vi "GetProbePlanCoordinates.vi"(8 "Use index as X coord":bool=TRUE, 9 "Probe Card Channels":i32=1) -> (0 "file path":string, 2 "OK?":bool, 3 "Array":T1(array[cluster]))   [LabVIEW 2018] (continued)
\nLabel=Strip\t101\tX=71108.80\ty=-38543.20 \nLabel=Strip\t102\tX=71464.66\ty=-38487.93 \nLabel=Strip\t103\tX=71121.99\ty=-38387.09 \nLabel=Strip\t104\tX=71477.83\ty=-38331.70 \nLabel=Strip\t105\tX=71135.13\ty=-38230.97 \nLabel=Strip\t106\tX=71490.95\ty=-38175.46 \nLabel=Strip\t107\tX=71148.21\ty=-38074.85 \nLabel=Strip\t108\tX=71504.01\ty=-38019.21 \nLabel=Strip\t109\tX=71161.24\ty=-37918.72 \nLabel=Strip\t110\tX=71517.02\ty=-37862.96 \nLabel=Strip\t111\tX=71174.22\ty=-37762.59 \nLabel=Strip\t112\tX=71529.98\ty=-37706.70 \nLabel=Strip\t113\tX=71187.14\ty=-37606.45 \nLabel=Strip\t114\tX=71542.88\ty=-37550.44 \nLabel=Strip\t115\tX=71200.01\ty=-37450.30 \nLabel=Strip\t116\tX=71555.73\ty=-37394.17 \nLabel=Strip\t117\tX=71212.82\ty=-37294.15 \nLabel=Strip\t118\tX=71568.53\ty=-37237.90 \nLabel=Strip\t119\tX=71225.59\ty=-37138.00 \nLabel=Strip\t120\tX=71581.27\ty=-37081.62 \nLabel=Strip\t121\tX=71238.29\ty=-36981.83 \nLabel=Strip\t122\tX=71593.96\ty=-36925.33 \nLabel=Strip\t123\tX=71250.95\ty=-36825.67 \nLabel=Strip\t124\tX=71606.60\ty=-36769.04 \nLabel=Strip\t125\tX=71263.55\ty=-36669.50 \nLabel=Strip\t126\tX=71619.18\ty=-36612.75 \nLabel=Strip\t127\tX=71276.10\ty=-36513.32 \nLabel=Strip\t128\tX=71631.71\ty=-36456.45 \nLabel=Strip\t129\tX=71288.59\ty=-36357.13 \nLabel=Strip\t130\tX=71644.18\ty=-36300.14 \nLabel=Strip\t131\tX=71301.04\ty=-36200.95 \nLabel=Strip\t132\tX=71656.61\ty=-36143.83 \nLabel=Strip\t133\tX=71313.42\ty=-36044.75 \nLabel=Strip\t134\tX=71668.98\ty=-35987.52 \nLabel=Strip\t135\tX=71325.76\ty=-35888.55 \nLabel=Strip\t136\tX=71681.29\ty=-35831.20 \nLabel=Strip\t137\tX=71338.04\ty=-35732.35 \nLabel=Strip\t138\tX=71693.55\ty=-35674.87 \nLabel=Strip\t139\tX=71350.27\ty=-35576.14 \nLabel=Strip\t140\tX=71705.76\ty=-35518.54 \nLabel=Strip\t141\tX=71362.44\ty=-35419.93 \nLabel=Strip\t142\tX=71717.91\ty=-35362.20 \nLabel=Strip\t143\tX=71374.56\ty=-35263.71 \nLabel=Strip\t144\tX=71730.01\ty=-35205.86 \nLabel=Strip\t145\tX=71386.63\ty=-35107.48 \nLabel=Strip\t146\tX=71742.06\ty=-35049.51 \nLabel=Strip\t147\tX=71398.64\ty=-34951.25 \nLabel=Strip\t148\tX=71754.06\ty=-34893.16 \nLabel=Strip\t149\tX=71410.60\ty=-34795.02 \nLabel=Strip\t150\tX=71766.00\ty=-34736.80 \nLabel=Strip\t151\tX=71422.51\ty=-34638.78 \nLabel=Strip\t152\tX=71777.88\ty=-34580.44 \nLabel=Strip\t153\tX=71434.36\ty=-34482.53 \nLabel=Strip\t154\tX=71789.71\ty=-34424.07 \nLabel=Strip\t155\tX=71446.16\ty=-34326.28 \nLabel=Strip\t156\tX=71801.49\ty=-34267.70 \nLabel=Strip\t157\tX=71457.91\ty=-34170.02 \nLabel=Strip\t158\tX=71813.22\ty=-34111.32 \nLabel=Strip\t159\tX=71469.60\ty=-34013.76 \nLabel=Strip\t160\tX=71824.89\ty=-33954.93 \nLabel=Strip\t161\tX=71481.24\ty=-33857.50 \nLabel=Strip\t162\tX=71836.51\ty=-33798.55 \nLabel=Strip\t163\tX=71492.82\ty=-33701.23 \nLabel=Strip\t164\tX=71848.08\ty=-33642.15 \nLabel=Strip\t165\tX=71504.36\ty=-33544.95 \nLabel=Strip\t166\tX=71859.59\ty=-33485.76 \nLabel=Strip\t167\tX=71515.83\ty=-33388.67 \nLabel=Strip\t168\tX=71871.05\ty=-33329.35 \nLabel=Strip\t169\tX=71527.26\ty=-33232.39 \nLabel=Strip\t170\tX=71882.45\ty=-33172.94 \nLabel=Strip\t171\tX=71538.63\ty=-33076.09 \nLabel=Strip\t172\tX=71893.80\ty=-33016.53 \nLabel=Strip\t173\tX=71549.95\ty=-32919.80 \nLabel=Strip\t174\tX=71905.10\ty=-32860.11 \nLabel=Strip\t175\tX=71561.21\ty=-32763.50 \nLabel=Strip\t176\tX=71916.34\ty=-32703.69 \nLabel=Strip\t177\tX=71572.42\ty=-32607.19 \nLabel=Strip\t178\tX=71927.53\ty=-32547.26 \nLabel=Strip\t179\tX=71583.58\ty=-32450.88 \nLabel=Strip\t180\tX=71938.67\ty=-32390.83 \nLabel=Strip\t181\tX=71594.68\ty=-32294.57 \nLabel=Strip\t182\tX=71949.75\ty=-32234.39 \nLabel=Strip\t183\tX=71605.73\ty=-32138.25 \nLabel=Strip\t184\tX=71960.78\ty=-32077.95 \nLabel=Strip\t185\tX=71616.73\ty=-31981.93 \nLabel=Strip\t186\tX=71971.76\ty=-31921.50 \nLabel=Strip\t187\tX=71627.67\ty=-31825.60 \nLabel=Strip\t188\tX=71982.68\ty=-31765.05 \nLabel=Strip\t189\tX=71638.56\ty=-31669.26 \nLabel=Strip\t190\tX=71993.55\ty=-31608.59 \nLabel=Strip\t191\tX=71649.40\ty=-31512.92 \nLabel=Strip\t192\tX=72004.36\ty=-31452.13 \nLabel=Strip\t193\tX=71660.18\ty=-31356.58 \nLabel=Strip\t194\tX=72015.13\ty=-31295.67 \nLabel=Strip\t195\tX=71670.91\ty=-31200.23 \nLabel=Strip\t196\tX=72025.83\ty=-31139.20 \nLabel=Strip\t197\tX=71681.58\ty=-31043.88 \nLabel=Strip\t198\tX=72036.49\ty=-30982.72 \nLabel=Strip\t199\tX=71692.21\ty=-30887.52 \nLabel=Strip\t200\tX=72047.09\ty=-30826.24 \nLabel=Strip\t201\tX=71702.77\ty=-30731.16 \nLabel=Strip\t202\tX=72057.64\ty=-30669.76 \nLabel=Strip\t203\tX=71713.29\ty=-30574.79 \nLabel=Strip\t204\tX=72068.13\ty=-30513.27 \nLabel=Strip\t205\tX=71723.75\ty=-30418.42 \nLabel=Strip\t206\tX=72078.57\ty=-30356.77 \nLabel=Strip\t207\tX=71734.16\ty=-30262.04 \nLabel=Strip\t208\tX=72088.96\ty=-30200.27 \nLabel=Strip\t209\tX=71744.51\ty=-30105.66 \nLabel=Strip\t210\tX=72099.29\ty=-30043.77 \nLabel=Strip\t211\tX=71754.81\ty=-29949.28 \nLabel=Strip\t212\tX=72109.57\ty=-29887.26 \nLabel=Strip\t213\tX=71765.06\ty=-29792.89 \nLabel=Strip\t214\tX=72119.79\ty=-29730.75 \nLabel=Strip\t215\tX=71775.25\ty=-29636.49 \nLabel=Strip\t216\tX=72129.96\ty=-29574.23 \nLabel=Strip\t217\tX=71785.39\ty=-29480.09 \nLabel=Strip\t218\tX=72140.08\ty=-29417.71 \nLabel=Strip\t219\tX=71795.48\ty=-29323.69 \nLabel=Strip\t220\tX=72150.15\ty=-29261.19 \nLabel=Strip\t221\tX=71805.51\ty=-29167.28 \nLabel=Strip\t222\tX=72160.16\ty=-29104.66 \nLabel=Strip\t223\tX=71815.49\ty=-29010.87 \nLabel=Strip\t224\tX=72170.11\ty=-28948.12 \nLabel=Strip\t225\tX=71825.41\ty=-28854.45 \nLabel=Strip\t226\tX=72180.02\ty=-28791.58 \nLabel=Strip\t227\tX=71835.28\ty=-28698.03 \nLabel=Strip\t228\tX=72189.87\ty=-28635.04 \nLabel=Strip\t229\tX=71845.10\ty=-28541.60 \nLabel=Strip\t230\tX=72199.67\ty=-28478.49 \nLabel=Strip\t231\tX=71854.87\ty=-28385.17 \nLabel=Strip\t232\tX=72209.41\ty=-28321.94 \nLabel=Strip\t233\tX=71864.58\ty=-28228.74 \nLabel=Strip\t234\tX=72219.10\ty=-28165.38 \nLabel=Strip\t235\tX=71874.23\ty=-28072.30 \nLabel=Strip\t236\tX=72228.73\ty=-28008.82 \nLabel=Strip\t237\tX=71883.84\ty=-27915.86 \nLabel=Strip\t238\tX=72238.31\ty=-27852.26 \nLabel=Strip\t239\tX=71893.39\ty=-27759.41 \nLabel=Strip\t240\tX=72247.84\ty=-27695.69 \nLabel=Strip\t241\tX=71902.88\ty=-27602.96 \nLabel=Strip\t242\tX=72257.32\ty=-27539.11 \nLabel=Strip\t243\tX=71912.33\ty=-27446.50 \nLabel=Strip\t244\tX=72266.74\ty=-27382.53 \nLabel=Strip\t245\tX=71921.72\ty=-27290.04 \nLabel=Strip\t246\tX=72276.10\ty=-27225.95 \nLabel=Strip\t247\tX=71931.05\ty=-27133.58 \nLabel=Strip\t248\tX=72285.42\ty=-27069.36 \nLabel=Strip\t249\tX=71940.33\ty=-26977.11 \nLabel=Strip\t250\tX=72294.68\ty=-26912.77 \nLabel=Strip\t251\tX=71949.56\ty=-26820.63 \nLabel=Strip\t252\tX=72303.88\ty=-26756.18 \nLabel=Strip\t253\tX=71958.74\ty=-26664.16 \nLabel=Strip\t254\tX=72313.04\ty=-26599.58 \nLabel=Strip\t255\tX=71967.86\ty=-26507.68 \nLabel=Strip\t256\tX=72322.14\ty=-26442.97 \nLabel=Strip\t257\tX=71976.93\ty=-26351.19 \nLabel=Strip\t258\tX=72331.18\ty=-26286.37 \nLabel=Strip\t259\tX=71985.94\ty=-26194.70 \nLabel=Strip\t260\tX=72340.17\ty=-26129.75 \nLabel=Strip\t261\tX=71994.90\ty=-26038.21 \nLabel=Strip\t262\tX=72349.11\ty=-25973.14 \nLabel=Strip\t263\tX=72003.81\ty=-25881.71 \nLabel=Strip\t264\tX=72357.99\ty=-25816.52 \nLabel=Strip\t265\tX=72012.66\ty=-25725.21 \nLabel=Strip\t266\tX=72366.82\ty=-25659.89 \nLabel=Strip\t267\tX=72021.46\ty=-25568.70 \nLabel=Strip\t268\tX=72375.60\ty=-25503.27 \nLabel=Strip\t269\tX=72030.20\ty=-25412.19 \nLabel=Strip\t270\tX=72384.32\ty=-25346.63 \nLabel=Strip\t271\tX=72038.89\ty=-25255.68 \nLabel=Strip\t272\tX=72392.99\ty=-25190.00 \nLabel=Strip\t273\tX=72047.53\ty=-25099.16 \nLabel=Strip\t274\tX=72401.61\ty=-25033.36 \nLabel=Strip\t275\tX=72056.12\ty=-24942.64 \nLabel=Strip\t276\tX=72410.17\ty=-24876.71 \nLabel=Strip\t277\tX=72064.65\ty=-24786.11 \nLabel=Strip\t278\tX=72418.68\ty=-24720.06 \nLabel=Strip\t279\tX=72073.13\ty=-24629.58 \nLabel=Strip\t280\tX=72427.13\ty=-24563.41 \nLabel=Strip\t281\tX=72081.55\ty=-24473.05 \nLabel=Strip\t282\tX=72435.54\ty=-24406.76 \nLabel=Strip\t283\tX=72089.92\ty=-24316.51 \nLabel=Strip\t284\tX=72443.88\ty=-24250.10 \nLabel=Strip\t285\tX=72098.24\ty=-24159.97 \nLabel=Strip\t286\tX=72452.18\ty=-24093.43 \nLabel=Strip\t287\tX=72106.50\ty=-24003.42 \nLabel=Strip\t288\tX=72460.42\ty=-23936.77 \nLabel=Strip\t289\tX=72114.71\ty=-23846.87 \nLabel=Strip\t290\tX=72468.60\ty=-23780.09 \nLabel=Strip\t291\tX=72122.86\ty=-23690.32 \nLabel=Strip\t292\tX=72476.74\ty=-23623.42 \nLabel=Strip\t293\tX=72130.97\ty=-23533.76 \nLabel=Strip\t294\tX=72484.81\ty=-23466.74 \nLabel=Strip\t295\tX=72139.01\ty=-23377.20 \nLabel=Strip\t296\tX=72492.84\ty=-23310.06 \nLabel=Strip\t297\tX=72147.01\ty=-23220.63 \nLabel=Strip\t298\tX=72500.81\ty=-23153.37 \nLabel=Strip\t299\tX=72154.95\ty=-23064.07 \nLabel=Strip\t300\tX=72508.73\ty=-22996.68 \nLabel=Strip\t301\tX=72162.84\ty=-22907.49 \nLabel=Strip\t302\tX=72516.59\ty=-22839.98 \nLabel=Strip\t303\tX=72170.67\ty=-22750.92 \nLabel=Strip\t304\tX=72524.40\ty=-22683.29 \nLabel=Strip\t305\tX=72178.45\ty=-22594.34 \nLabel=Strip\t306\tX=72532.16\ty=-22526.58 \nLabel=Strip\t307\tX=72186.17\ty=-22437.75 \nLabel=Strip\t308\tX=72539.86\ty=-22369.88 \nLabel=Strip\t309\tX=72193.85\ty=-22281.17 \nLabel=Strip\t310\tX=72547.51\ty=-22213.17 \nLabel=Strip\t311\tX=72201.47\ty=-22124.58 \nLabel=Strip\t312\tX=72555.11\ty=-22056.46 \nLabel=Strip\t313\tX=72209.03\ty=-21967.98 \nLabel=Strip\t314\tX=72562.65\ty=-21899.74 \nLabel=Strip\t315\tX=72216.54\ty=-21811.38 \nLabel=Strip\t316\tX=72570.14\ty=-21743.02 \nLabel=Strip\t317\tX=72224.00\ty=-21654.78 \nLabel=Strip\t318\tX=72577.57\ty=-21586.30 \nLabel=Strip\t319\tX=72231.40\ty=-21498.18 \nLabel=Strip\t320\tX=72584.95\ty=-21429.57 \nLabel=Strip\t321\tX=72238.75\ty=-21341.57 \nLabel=Strip\t322\tX=72592.28\ty=-21272.84 \nLabel=Strip\t323\tX=72246.05\ty=-21184.96 \nLabel=Strip\t324\tX=72599.55\ty=-21116.11 \nLabel=Strip\t325\tX=72253.29\ty=-21028.34 \nLabel=Strip\t326\tX=72606.77\ty=-20959.37 \nLabel=Strip\t327\tX=72260.48\ty=-20871.72 \nLabel=Strip\t328\tX=72613.94\ty=-20802.63 \nLabel=Strip\t329\tX=72267.62\ty=-20715.10 \nLabel=Strip\t330\tX=72621.05\ty=-20645.88 \nLabel=Strip\t331\tX=72274.70\ty=-20558.47 \nLabel=Strip\t332\tX=72628.11\ty=-20489.13 \nLabel=Strip\t333\tX=72281.73\ty=-20401.84 \nLabel=Strip\t334\tX=72635.11\ty=-20332.38 \nLabel=Strip\t335\tX=72288.70\ty=-20245.21 \nLabel=Strip\t336\tX=72642.06\ty=-20175.63 \nLabel=Strip\t337\tX=72295.62\ty=-20088.57 \nLabel=Strip\t338\tX=72648.96\ty=-20018.87 \nLabel=Strip\t339\tX=72302.49\ty=-19931.93 \nLabel=Strip\t340\tX=72655.80\ty=-19862.11 \nLabel=Strip\t341\tX=72309.30\ty=-19775.29 \nLabel=Strip\t342\tX=72662.59\ty=-19705.34 \nLabel=Strip\t343\tX=72316.06\ty=-19618.64 \nLabel=Strip\t344\tX=72669.33\ty=-19548.57 \nLabel=Strip\t345\tX=72322.77\ty=-19461.99 \nLabel=Strip\t346\tX=72676.01\ty=-19391.80 \nLabel=Strip\t347\tX=72329.42\ty=-19305.34 \nLabel=Strip\t348\tX=72682.63\ty=-19235.03 \nLabel=Strip\t349\tX=72336.02\ty=-19148.68 \nLabel=Strip\t350\tX=72689.21\ty=-19078.25 \nLabel=Strip\t351\tX=72342.56\ty=-18992.02 \nLabel=Strip\t352\tX=72695.73\ty=-18921.47 \nLabel=Strip\t353\tX=72349.06\ty=-18835.36 \nLabel=Strip\t354\tX=72702.20\ty=-18764.68 \nLabel=Strip\t355\tX=72355.49\ty=-18678.69 \nLabel=Strip\t356\tX=72708.61\ty=-18607.89 \nLabel=Strip\t357\tX=72361.88\ty=-18522.02 \nLabel=Strip\t358\tX=72714.97\ty=-18451.10 \nLabel=Strip\t359\tX=72368.21\ty=-18365.35 \nLabel=Strip\t360\tX=72721.27\ty=-18294.31 \nLabel=Strip\t361\tX=72374.48\ty=-18208.67 \nLabel=Strip\t362\tX=72727.53\ty=-18137.51 \nLabel=Strip\t363\tX=72380.70\ty=-18051.99 \nLabel=Strip\t364\tX=72733.72\ty=-17980.71 \nLabel=Strip\t365\tX=72386.87\ty=-17895.31 \nLabel=Strip\t366\tX=72739.87\ty=-17823.90 \nLabel=Strip\t367\tX=72392.99\ty=-17738.63 \nLabel=Strip\t368\tX=72745.96\ty=-17667.10 \nLabel=Strip\t369\tX=72399.05\ty=-17581.94 \nLabel=Strip\t370\tX=72751.99\ty=-17510.28 \nLabel=Strip\t371\tX=72405.06\ty=-17425.25 \nLabel=Strip\t372\tX=72757.98\ty=-17353.47 \nLabel=Strip\t373\tX=72411.01\ty=-17268.55 \nLabel=Strip\t374\tX=72763.91\ty=-17196.65 \nLabel=Strip\t375\tX=72416.91\ty=-17111.85 \nLabel=Strip\t376\tX=72769.78\ty=-17039.84 \nLabel=Strip\t377\tX=72422.76\ty=-16955.15 \nLabel=Strip\t378\tX=72775.60\ty=-16883.01 \nLabel=Strip\t379\tX=72428.55\ty=-16798.45 \nLabel=Strip\t380\tX=72781.37\ty=-16726.19 \nLabel=Strip\t381\tX=72434.29\ty=-16641.74 \nLabel=Strip\t382\tX=72787.09\ty=-16569.36 \nLabel=Strip\t383\tX=72439.97\ty=-16485.03 \nLabel=Strip\t384\tX=72792.74\ty=-16412.53 \nLabel=Strip\t385\tX=72445.60\ty=-16328.32 \nLabel=Strip\t386\tX=72798.35\ty=-16255.69 \nLabel=Strip\t387\tX=72451.18\ty=-16171.60 \nLabel=Strip\t388\tX=72803.90\ty=-16098.85 \nLabel=Strip\t389\tX=72456.70\ty=-16014.88 \nLabel=Strip\t390\tX=72809.40\ty=-15942.01 \nLabel=Strip\t391\tX=72462.17\ty=-15858.16 \nLabel=Strip\t392\tX=72814.85\ty=-15785.17 \nLabel=Strip\t393\tX=72467.59\ty=-15701.44 \nLabel=Strip\t394\tX=72820.24\ty=-15628.32 \nLabel=Strip\t395\tX=72472.95\ty=-15544.71 \nLabel=Strip\t396\tX=72825.58\ty=-15471.47 \nLabel=Strip\t397\tX=72478.26\ty=-15387.98 \nLabel=Strip\t398\tX=72830.86\ty=-15314.62 \nLabel=Strip\t399\tX=72483.52\ty=-15231.24 \nLabel=Strip\t400\tX=72836.09\ty=-15157.77 \nLabel=Strip\t401\tX=72488.72\ty=-15074.51 \nLabel=Strip\t402\tX=72841.27\ty=-15000.91 \nLabel=Strip\t403\tX=72493.86\ty=-14917.77 \nLabel=Strip\t404\tX=72846.39\ty=-14844.05 \nLabel=Strip\t405\tX=72498.96\ty=-14761.03 \nLabel=Strip\t406\tX=72851.46\ty=-14687.18 \nLabel=Strip\t407\tX=72504.00\ty=-14604.28 \nLabel=Strip\t408\tX=72856.47\ty=-14530.32 \nLabel=Strip\t409\tX=72508.98\ty=-14447.53 \nLabel=Strip\t410\tX=72861.43\ty=-14373.45 \nLabel=Strip\t411\tX=72513.92\ty=-14290.78 \nLabel=Strip\t412\tX=72866.34\ty=-14216.58 \nLabel=Strip\t413\tX=72518.79\ty=-14134.03 \nLabel=Strip\t414\tX=72871.19\ty=-14059.70 \nLabel=Strip\t415\tX=72523.62\ty=-13977.28 \nLabel=Strip\t416\tX=72875.99\ty=-13902.83 \nLabel=Strip\t417\tX=72528.39\ty=-13820.52 \nLabel=Strip\t418\tX=72880.74\ty=-13745.95 \nLabel=Strip\t419\tX=72533.11\ty=-13663.76 \nLabel=Strip\t420\tX=72885.43\ty=-13589.07 \nLabel=Strip\t421\tX=72537.77\ty=-13506.99 \nLabel=Strip\t422\tX=72890.06\ty=-13432.18 \nLabel=Strip\t423\tX=72542.38\ty=-13350.23 \nLabel=Strip\t424\tX=72894.65\ty=-13275.29 \nLabel=Strip\t425\tX=72546.94\ty=-13193.46 \nLabel=Strip\t426\tX=72899.18\ty=-13118.40 \nLabel=Strip\t427\tX=72551.44\ty=-13036.69 \nLabel=Strip\t428\tX=72903.65\ty=-12961.51 \nLabel=Strip\t429\tX=72555.89\ty=-12879.91 \nLabel=Strip\t430\tX=72908.08\ty=-12804.61 \nLabel=Strip\t431\tX=72560.28\ty=-12723.14 \nLabel=Strip\t432\tX=72912.45\ty=-12647.72 \nLabel=Strip\t433\tX=72564.62\ty=-12566.36 \nLabel=Strip\t434\tX=72916.76\ty=-12490.82 \nLabel=Strip\t435\tX=72568.91\ty=-12409.58 \nLabel=Strip\t436\tX=72921.02\ty=-12333.91 \nLabel=Strip\t437\tX=72573.14\ty=-12252.79 \nLabel=Strip\t438\tX=72925.23\ty=-12177.01 \nLabel=Strip\t439\tX=72577.32\ty=-12096.01 \nLabel=Strip\t440\tX=72929.38\ty=-12020.10 \nLabel=Strip\t441\tX=72581.45\ty=-11939.22 \nLabel=Strip\t442\tX=72933.48\ty=-11863.19 \nLabel=Strip\t443\tX=72585.52\ty=-11782.43 \nLabel=Strip\t444\tX=72937.53\ty=-11706.28 \nLabel=Strip\t445\tX=72589.54\ty=-11625.63 \nLabel=Strip\t446\tX=72941.52\ty=-11549.36 \nLabel=Strip\t447\tX=72593.50\ty=-11468.84 \nLabel=Strip\t448\tX=72945.46\ty=-11392.44 \nLabel=Strip\t449\tX=72597.41\ty=-11312.04 \nLabel=Strip\t450\tX=72949.34\ty=-11235.52 \nLabel=Strip\t451\tX=72601.27\ty=-11155.24 \nLabel=Strip\t452\tX=72953.17\ty=-11078.60 \nLabel=Strip\t453\tX=72605.07\ty=-10998.43 \nLabel=Strip\t454\tX=72956.95\ty=-10921.68 \nLabel=Strip\t455\tX=72608.82\ty=-10841.63 \nLabel=Strip\t456\tX=72960.67\ty=-10764.10 \nLabel=Strip\t457\tX=72612.51\ty=-10684.54 \nLabel=Strip\t458\tX=72964.34\ty=-10607.43 \nLabel=Strip\t459\tX=72616.16\ty=-10527.87 \nLabel=Strip\t460\tX=72967.95\ty=-10450.76 \nLabel=Strip\t461\tX=72619.74\ty=-10371.20 \nLabel=Strip\t462\tX=72971.51\ty=-10294.08 \nLabel=Strip\t463\tX=72623.28\ty=-10214.52 \nLabel=Strip\t464\tX=72975.02\ty=-10137.41 \nLabel=Strip\t465\tX=72626.76\ty=-10057.85 \nLabel=Strip\t466\tX=72978.47\ty=-9980.73 \nLabel=Strip\t467\tX=72630.18\ty=-9900.75 \nLabel=Strip\t468\tX=72981.87\ty=-9823.14 \nLabel=Strip\t469\tX=72633.55\ty=-9743.92 \nLabel=Strip\t470\tX=72985.22\ty=-9666.20 \nLabel=Strip\t471\tX=72636.87\ty=-9587.10 \nLabel=Strip\t472\tX=72988.51\ty=-9509.25 \nLabel=Strip\t473\tX=72640.14\ty=-9430.27 \nLabel=Strip\t474\tX=72991.75\ty=-9352.31 \nLabel=Strip\t475\tX=72643.35\ty=-9273.45 \nLabel=Strip\t476\tX=72994.93\ty=-9195.36 \nLabel=Strip\t477\tX=72646.51\ty=-9116.62 \nLabel=Strip\t478\tX=72998.06\ty=-9038.40 \nLabel=Strip\t479\tX=72649.61\ty=-8959.79 \nLabel=Strip\t480\tX=73001.14\ty=-8881.45 \nLabel=Strip\t481\tX=72652.66\ty=-8802.95 \nLabel=Strip\t482\tX=73004.16\ty=-8724.50 \nLabel=Strip\t483\tX=72655.65\ty=-8646.11 \nLabel=Strip\t484\tX=73007.13\ty=-8567.54 \nLabel=Strip\t485\tX=72658.59\ty=-8489.28 \nLabel=Strip\t486\tX=73010.04\ty=-8410.58 \nLabel=Strip\t487\tX=72661.48\ty=-8332.43 \nLabel=Strip\t488\tX=73012.91\ty=-8253.62 \nLabel=Strip\t489\tX=72664.32\ty=-8175.59 \nLabel=Strip\t490\tX=73015.71\ty=-8096.65 \nLabel=Strip\t491\tX=72667.10\ty=-8018.75 \nLabel=Strip\t492\tX=73018.47\ty=-7939.69 \nLabel=Strip\t493\tX=72669.82\ty=-7861.90 \nLabel=Strip\t494\tX=73021.17\ty=-7782.72 \nLabel=Strip\t495\tX=72672.50\ty=-7705.05 \nLabel=Strip\t496\tX=73023.81\ty=-7625.75 \nLabel=Strip\t497\tX=72675.11\ty=-7548.20 \nLabel=Strip\t498\tX=73026.40\ty=-7468.78 \nLabel=Strip\t499\tX=72677.68\ty=-7391.35 \nLabel=Strip\t500\tX=73028.94\ty=-7311.81 \nLabel=Strip\t501\tX=72680.19\ty=-7234.50 \nLabel=Strip\t502\tX=73031.42\ty=-7154.83 \nLabel=Strip\t503\tX=72682.65\ty=-7077.64 \nLabel=Strip\t504\tX=73033.85\ty=-6997.85 \nLabel=Strip\t505\tX=72685.05\ty=-6920.78 \nLabel=Strip\t506\tX=73036.23\ty=-6840.87 \nLabel=Strip\t507\tX=72687.40\ty=-6763.92 \nLabel=Strip\t508\tX=73038.55\ty=-6683.89 \nLabel=Strip\t509\tX=72689.70\ty=-6607.06 \nLabel=Strip\t510\tX=73040.82\ty=-6526.91 \nLabel=Strip\t511\tX=72691.94\ty=-6450.20 \nLabel=Strip\t512\tX=73043.03\ty=-6369.93 \nLabel=Strip\t513\tX=72694.13\ty=-6293.33 \nLabel=Strip\t514\tX=73045.19\ty=-6212.94 \nLabel=Strip\t515\tX=72696.26\ty=-6136.47 \nLabel=Strip\t516\tX=73047.30\ty=-6055.95 \nLabel=Strip\t517\tX=72698.34\ty=-5979.60 \nLabel=Strip\t518\tX=73049.35\ty=-5898.96 \nLabel=Strip\t519\tX=72700.37\ty=-5822.73 \nLabel=Strip\t520\tX=73051.35\ty=-5741.97 \nLabel=Strip\t521\tX=72702.34\ty=-5665.86 \nLabel=Strip\t522\tX=73053.30\ty=-5584.98 \nLabel=Strip\t523\tX=72704.26\ty=-5508.98 \nLabel=Strip\t524\tX=73055.19\ty=-5427.98 \nLabel=Strip\t525\tX=72706.12\ty=-5352.11 \nLabel=Strip\t526\tX=73057.02\ty=-5270.99 \nLabel=Strip\t527\tX=72707.93\ty=-5195.23 \nLabel=Strip\t528\tX=73058.81\ty=-5113.99 \nLabel=Strip\t529\tX=72709.69\ty=-5038.35 \nLabel=Strip\t530\tX=73060.54\ty=-4956.99 \nLabel=Strip\t531\tX=72711.39\ty=-4881.47 \nLabel=Strip\t532\tX=73062.21\ty=-4799.99 \nLabel=Strip\t533\tX=72713.04\ty=-4724.59 \nLabel=Strip\t534\tX=73063.83\ty=-4642.98 \nLabel=Strip\t535\tX=72714.64\ty=-4567.70 \nLabel=Strip\t536\tX=73065.40\ty=-4485.98 \nLabel=Strip\t537\tX=72716.18\ty=-4410.82 \nLabel=Strip\t538\tX=73066.91\ty=-4328.97 \nLabel=Strip\t539\tX=72717.67\ty=-4253.93 \nLabel=Strip\t540\tX=73068.37\ty=-4171.97 \nLabel=Strip\t541\tX=72719.10\ty=-4097.04 \nLabel=Strip\t542\tX=73069.78\ty=-4014.96 \nLabel=Strip\t543\tX=72720.48\ty=-3940.15 \nLabel=Strip\t544\tX=73071.13\ty=-3857.95 \nLabel=Strip\t545\tX=72721.81\ty=-3783.26 \nLabel=Strip\t546\tX=73072.43\ty=-3700.93 \nLabel=Strip\t547\tX=72723.08\ty=-3626.37 \nLabel=Strip\t548\tX=73073.67\ty=-3543.92 \nLabel=Strip\t549\tX=72724.30\ty=-3469.47 \nLabel=Strip\t550\tX=73074.86\ty=-3386.90 \nLabel=Strip\t551\tX=72725.46\ty=-3312.58 \nLabel=Strip\t552\tX=73076.00\ty=-3229.89 \nLabel=Strip\t553\tX=72726.57\ty=-3155.68 \nLabel=Strip\t554\tX=73077.08\ty=-3072.87 \nLabel=Strip\t555\tX=72727.63\ty=-2998.78 \nLabel=Strip\t556\tX=73078.11\ty=-2915.85 \nLabel=Strip\t557\tX=72728.63\ty=-2841.88 \nLabel=Strip\t558\tX=73079.08\ty=-2758.83 \nLabel=Strip\t559\tX=72729.58\ty=-2684.98 \nLabel=Strip\t560\tX=73080.00\ty=-2601.81 \nLabel=Strip\t561\tX=72730.48\ty=-2528.08 \nLabel=Strip\t562\tX=73080.87\ty=-2444.78 \nLabel=Strip\t563\tX=72731.32\ty=-2371.17 \nLabel=Strip\t564\tX=73081.68\ty=-2287.76 \nLabel=Strip\t565\tX=72732.11\ty=-2214.27 \nLabel=Strip\t566\tX=73082.44\ty=-2130.73 \nLabel=Strip\t567\tX=72732.84\ty=-2057.36 \nLabel=Strip\t568\tX=73083.15\ty=-1973.70 \nLabel=Strip\t569\tX=72733.52\ty=-1900.45 \nLabel=Strip\t570\tX=73083.80\ty=-1816.68 \nLabel=Strip\t571\tX=72734.14\ty=-1743.55 \nLabel=Strip\t572\tX=73084.39\ty=-1659.65 \nLabel=Strip\t573\tX=72734.72\ty=-1586.64 \nLabel=Strip\t574\tX=73084.94\ty=-1502.61 \nLabel=Strip\t575\tX=72735.23\ty=-1429.72 \nLabel=Strip\t576\tX=73085.43\ty=-1345.58 \nLabel=Strip\t577\tX=72735.70\ty=-1272.81 \nLabel=Strip\t578\tX=73085.86\ty=-1188.55 \nLabel=Strip\t579\tX=72736.11\ty=-1115.90 \nLabel=Strip\t580\tX=73086.24\ty=-1031.51 \nLabel=Strip\t581\tX=72736.46\ty=-958.98 \nLabel=Strip\t582\tX=73086.57\ty=-874.48 \nLabel=Strip\t583\tX=72736.77\ty=-802.07 \nLabel=Strip\t584\tX=73086.84\ty=-717.44 \nLabel=Strip\t585\tX=72737.02\ty=-645.15 \nLabel=Strip\t586\tX=73087.06\ty=-560.40 \nLabel=Strip\t587\tX=72737.21\ty=-488.23 \nLabel=Strip\t588\tX=73087.23\ty=-403.36 \nLabel=Strip\t589\tX=72737.35\ty=-331.31 \nLabel=Strip\t590\tX=73087.34\ty=-246.32 \nLabel=Strip\t591\tX=72737.44\ty=-174.39 \nLabel=Strip\t592\tX=73087.40\ty=-89.28 \nLabel=Strip\t593\tX=72737.47\ty=-17.47 \nLabel=Strip\t594\tX=73087.40\ty=67.76 \nLabel=Strip\t595\tX=72737.45\ty=139.46 \nLabel=Strip\t596\tX=73087.35\ty=224.80 \nLabel=Strip\t597\tX=72737.38\ty=296.38 \nLabel=Strip\t598\tX=73087.25\ty=381.85 \nLabel=Strip\t599\tX=72737.25\ty=453.31 \nLabel=Strip\t600\tX=73087.09\ty=538.89 \nLabel=Strip\t601\tX=72737.06\ty=610.23 \nLabel=Strip\t602\tX=73086.88\ty=695.94 \nLabel=Strip\t603\tX=72736.83\ty=767.16 \nLabel=Strip\t604\tX=73086.61\ty=852.99 \nLabel=Strip\t605\tX=72736.54\ty=924.09 \nLabel=Strip\t606\tX=73086.29\ty=1010.04 \nLabel=Strip\t607\tX=72736.19\ty=1081.01 \nLabel=Strip\t608\tX=73085.92\ty=1167.09 \nLabel=Strip\t609\tX=72735.79\ty=1237.94 \nLabel=Strip\t610\tX=73085.49\ty=1324.14 \nLabel=Strip\t611\tX=72735.34\ty=1394.87 \nLabel=Strip\t612\tX=73085.01\ty=1481.19 \nLabel=Strip\t613\tX=72734.84\ty=1551.81 \nLabel=Strip\t614\tX=73084.47\ty=1638.24 \nLabel=Strip\t615\tX=72734.28\ty=1708.74 \nLabel=Strip\t616\tX=73083.88\ty=1795.29 \nLabel=Strip\t617\tX=72733.66\ty=1865.67 \nLabel=Strip\t618\tX=73083.24\ty=1952.35 \nLabel=Strip\t619\tX=72733.00\ty=2022.60 \nLabel=Strip\t620\tX=73082.54\ty=2109.40 \nLabel=Strip\t621\tX=72732.27\ty=2179.54 \nLabel=Strip\t622\tX=73081.79\ty=2266.45 \nLabel=Strip\t623\tX=72731.50\ty=2336.47 \nLabel=Strip\t624\tX=73080.98\ty=2423.51 \nLabel=Strip\t625\tX=72730.67\ty=2493.41 \nLabel=Strip\t626\tX=73080.13\ty=2580.57 \nLabel=Strip\t627\tX=72729.78\ty=2650.35 \nLabel=Strip\t628\tX=73079.21\ty=2737.62 \nLabel=Strip\t629\tX=72728.85\ty=2807.29 \nLabel=Strip\t630\tX=73078.24\ty=2894.68 \nLabel=Strip\t631\tX=72727.86\ty=2964.22 \nLabel=Strip\t632\tX=73077.22\ty=3051.74 \nLabel=Strip\t633\tX=72726.81\ty=3121.16 \nLabel=Strip\t634\tX=73076.15\ty=3208.80 \nLabel=Strip\t635\tX=72725.71\ty=3278.10 \nLabel=Strip\t636\tX=73075.02\ty=3365.86 \nLabel=Strip\t637\tX=72724.56\ty=3435.04 \nLabel=Strip\t638\tX=73073.84\ty=3522.92 \nLabel=Strip\t639\tX=72723.35\ty=3591.98 \nLabel=Strip\t640\tX=73072.60\ty=3679.98 \nLabel=Strip\t641\tX=72722.09\ty=3748.93 \nLabel=Strip\t642\tX=73071.31\ty=3837.05 \nLabel=Strip\t643\tX=72720.78\ty=3905.87 \nLabel=Strip\t644\tX=73069.96\ty=3994.11 \nLabel=Strip\t645\tX=72719.41\ty=4062.81 \nLabel=Strip\t646\tX=73068.56\ty=4151.17 \nLabel=Strip\t647\tX=72717.99\ty=4219.75 \nLabel=Strip\t648\tX=73067.11\ty=4308.23 \nLabel=Strip\t649\tX=72716.51\ty=4376.70 \nLabel=Strip\t650\tX=73065.60\ty=4465.30 \nLabel=Strip\t651\tX=72714.98\ty=4533.64 \nLabel=Strip\t652\tX=73064.04\ty=4622.36 \nLabel=Strip\t653\tX=72713.39\ty=4690.59 \nLabel=Strip\t654\tX=73062.43\ty=4779.43 \nLabel=Strip\t655\tX=72711.76\ty=4847.53 \nLabel=Strip\t656\tX=73060.76\ty=4936.49 \nLabel=Strip\t657\tX=72710.06\ty=5004.48 \nLabel=Strip\t658\tX=73059.04\ty=5093.56 \nLabel=Strip\t659\tX=72708.32\ty=5161.42 \nLabel=Strip\t660\tX=73057.26\ty=5250.63 \nLabel=Strip\t661\tX=72706.52\ty=5318.37 \nLabel=Strip\t662\tX=73055.43\ty=5407.69 \nLabel=Strip\t663\tX=72704.66\ty=5475.32 \nLabel=Strip\t664\tX=73053.54\ty=5564.76 \nLabel=Strip\t665\tX=72702.76\ty=5632.27 \nLabel=Strip\t666\tX=73051.61\ty=5721.83 \nLabel=Strip\t667\tX=72700.79\ty=5789.21 \nLabel=Strip\t668\tX=73049.61\ty=5878.90 \nLabel=Strip\t669\tX=72698.78\ty=5946.16 \nLabel=Strip\t670\tX=73047.57\ty=6035.97 \nLabel=Strip\t671\tX=72696.71\ty=6103.11 \nLabel=Strip\t672\tX=73045.47\ty=6193.04 \nLabel=Strip\t673\tX=72694.58\ty=6260.06 \nLabel=Strip\t674\tX=73043.31\ty=6350.10 \nLabel=Strip\t675\tX=72692.41\ty=6417.01 \nLabel=Strip\t676\tX=73041.10\ty=6507.17 \nLabel=Strip\t677\tX=72690.18\ty=6573.96 \nLabel=Strip\t678\tX=73038.84\ty=6664.24 \nLabel=Strip\t679\tX=72687.89\ty=6730.91 \nLabel=Strip\t680\tX=73036.52\ty=6821.31 \nLabel=Strip\t681\tX=72685.55\ty=6887.86 \nLabel=Strip\t682\tX=73034.15\ty=6978.38 \nLabel=Strip\t683\tX=72683.16\ty=7044.81 \nLabel=Strip\t684\tX=73031.73\ty=7135.45 \nLabel=Strip\t685\tX=72680.71\ty=7201.76 \nLabel=Strip\t686\tX=73029.25\ty=7292.52 \nLabel=Strip\t687\tX=72678.21\ty=7358.71 \nLabel=Strip\t688\tX=73026.72\ty=7449.59 \nLabel=Strip\t689\tX=72675.65\ty=7515.66 \nLabel=Strip\t690\tX=73024.13\ty=7606.67 \nLabel=Strip\t691\tX=72673.04\ty=7672.61 \nLabel=Strip\t692\tX=73021.49\ty=7763.74 \nLabel=Strip\t693\tX=72670.38\ty=7829.56 \nLabel=Strip\t694\tX=73018.80\ty=7920.81 \nLabel=Strip\t695\tX=72667.67\ty=7986.51 \nLabel=Strip\t696\tX=73016.05\ty=8077.88 \nLabel=Strip\t697\tX=72664.89\ty=8143.46 \nLabel=Strip\t698\tX=73013.25\ty=8234.95 \nLabel=Strip\t699\tX=72662.07\ty=8300.41 \nLabel=Strip\t700\tX=73010.39\ty=8392.02 \nLabel=Strip\t701\tX=72659.19\ty=8457.36 \nLabel=Strip\t702\tX=73007.48\ty=8549.09 \nLabel=Strip\t703\tX=72656.26\ty=8614.32 \nLabel=Strip\t704\tX=73004.52\ty=8706.16 \nLabel=Strip\t705\tX=72653.27\ty=8771.27 \nLabel=Strip\t706\tX=73001.50\ty=8863.24 \nLabel=Strip\t707\tX=72650.23\ty=8928.22 \nLabel=Strip\t708\tX=72998.42\ty=9020.31 \nLabel=Strip\t709\tX=72647.14\ty=9085.17 \nLabel=Strip\t710\tX=72995.30\ty=9177.38 \nLabel=Strip\t711\tX=72643.99\ty=9242.12 \nLabel=Strip\t712\tX=72992.12\ty=9334.45 \nLabel=Strip\t713\tX=72640.78\ty=9399.07 \nLabel=Strip\t714\tX=72988.88\ty=9491.52 \nLabel=Strip\t715\tX=72637.53\ty=9556.02 \nLabel=Strip\t716\tX=72985.60\ty=9648.59 \nLabel=Strip\t717\tX=72634.22\ty=9712.97 \nLabel=Strip\t718\tX=72982.25\ty=9805.66 \nLabel=Strip\t719\tX=72630.85\ty=9869.92 \nLabel=Strip\t720\tX=72978.86\ty=9962.73 \nLabel=Strip\t721\tX=72627.43\ty=10026.88 \nLabel=Strip\t722\tX=72975.41\ty=10119.81 \nLabel=Strip\t723\tX=72623.96\ty=10183.83 \nLabel=Strip\t724\tX=72971.90\ty=10276.88 \nLabel=Strip\t725\tX=72620.44\ty=10340.78 \nLabel=Strip\t726\tX=72968.34\ty=10433.95 \nLabel=Strip\t727\tX=72616.86\ty=10497.73 \nLabel=Strip\t728\tX=72964.73\ty=10591.02 \nLabel=Strip\t729\tX=72613.22\ty=10654.68 \nLabel=Strip\t730\tX=72961.07\ty=10748.09 \nLabel=Strip\t731\tX=72609.53\ty=10811.63 \nLabel=Strip\t732\tX=72957.35\ty=10905.16 \nLabel=Strip\t733\tX=72605.79\ty=10968.58 \nLabel=Strip\t734\tX=72953.57\ty=11062.23 \nLabel=Strip\t735\tX=72602.00\ty=11125.53 \nLabel=Strip\t736\tX=72949.74\ty=11219.29 \nLabel=Strip\t737\tX=72598.15\ty=11282.48 \nLabel=Strip\t738\tX=72945.86\ty=11376.36 \nLabel=Strip\t739\tX=72594.24\ty=11439.42 \nLabel=Strip\t740\tX=72941.93\ty=11533.43 \nLabel=Strip\t741\tX=72590.28\ty=11596.37 \nLabel=Strip\t742\tX=72937.94\ty=11690.50 \nLabel=Strip\t743\tX=72586.27\ty=11753.32 \nLabel=Strip\t744\tX=72933.89\ty=11847.57 \nLabel=Strip\t745\tX=72582.21\ty=11910.27 \nLabel=Strip\t746\tX=72929.79\ty=12004.64 \nLabel=Strip\t747\tX=72578.09\ty=12067.22 \nLabel=Strip\t748\tX=72925.64\ty=12161.70 \nLabel=Strip\t749\tX=72573.91\ty=12224.16 \nLabel=Strip\t750\tX=72921.43\ty=12318.77 \nLabel=Strip\t751\tX=72569.69\ty=12381.11 \nLabel=Strip\t752\tX=72917.17\ty=12475.84 \nLabel=Strip\t753\tX=72565.41\ty=12538.06 \nLabel=Strip\t754\tX=72912.86\ty=12632.90 \nLabel=Strip\t755\tX=72561.07\ty=12695.00 \nLabel=Strip\t756\tX=72908.49\ty=12789.97 \nLabel=Strip\t757\tX=72556.68\ty=12851.95 \nLabel=Strip\t758\tX=72904.07\ty=12947.03 \nLabel=Strip\t759\tX=72552.24\ty=13008.89 \nLabel=Strip\t760\tX=72899.59\ty=13104.10 \nLabel=Strip\t761\tX=72547.74\ty=13165.84 \nLabel=Strip\t762\tX=72895.06\ty=13261.16 \nLabel=Strip\t763\tX=72543.19\ty=13322.78 \nLabel=Strip\t764\tX=72890.48\ty=13418.23 \nLabel=Strip\t765\tX=72538.58\ty=13479.72 \nLabel=Strip\t766\tX=72885.84\ty=13575.29 \nLabel=Strip\t767\tX=72533.92\ty=13636.67 \nLabel=Strip\t768\tX=72881.15\ty=13732.35 \nLabel=Strip\t769\tX=72529.21\ty=13793.61 \nLabel=Strip\t770\tX=72876.40\ty=13889.41 \nLabel=Strip\t771\tX=72524.44\ty=13950.55 \nLabel=Strip\t772\tX=72871.60\ty=14046.47 \nLabel=Strip\t773\tX=72519.62\ty=14107.49 \nLabel=Strip\t774\tX=72866.75\ty=14203.53 \nLabel=Strip\t775\tX=72514.75\ty=14264.43 \nLabel=Strip\t776\tX=72861.84\ty=14360.59 \nLabel=Strip\t777\tX=72509.82\ty=14421.37 \nLabel=Strip\t778\tX=72856.88\ty=14517.65 \nLabel=Strip\t779\tX=72504.83\ty=14578.31 \nLabel=Strip\t780\tX=72851.86\ty=14674.71 \nLabel=Strip\t781\tX=72499.80\ty=14735.25 \nLabel=Strip\t782\tX=72846.79\ty=14831.77 \nLabel=Strip\t783\tX=72494.71\ty=14892.18 \nLabel=Strip\t784\tX=72841.67\ty=14988.83 \nLabel=Strip\t785\tX=72489.56\ty=15049.12 \nLabel=Strip\t786\tX=72836.49\ty=15145.88 \nLabel=Strip\t787\tX=72484.36\ty=15206.06 \nLabel=Strip\t788\tX=72831.26\ty=15302.94 \nLabel=Strip\t789\tX=72479.11\ty=15362.99 \nLabel=Strip\t790\tX=72825.97\ty=15459.99 \nLabel=Strip\t791\tX=72473.80\ty=15519.93 \nLabel=Strip\t792\tX=72820.63\ty=15617.05 \nLabel=Strip\t793\tX=72468.44\ty=15676.86 \nLabel=Strip\t794\tX=72815.24\ty=15774.10 \nLabel=Strip\t795\tX=72463.03\ty=15833.79 \nLabel=Strip\t796\tX=72809.79\ty=15931.15 \nLabel=Strip\t797\tX=72457.56\ty=15990.72 \nLabel=Strip\t798\tX=72804.29\ty=16088.21 \nLabel=Strip\t799\tX=72452.03\ty=16147.66 \nLabel=Strip\t800\tX=72798.73\ty=16245.26 \nLabel=Strip\t801\tX=72446.46\ty=16304.59 \nLabel=Strip\t802\tX=72793.12\ty=16402.31 \nLabel=Strip\t803\tX=72440.83\ty=16461.52 \nLabel=Strip\t804\tX=72787.45\ty=16559.36 \nLabel=Strip\t805\tX=72435.14\ty=16618.44 \nLabel=Strip\t806\tX=72781.74\ty=16716.40 \nLabel=Strip\t807\tX=72429.40\ty=16775.37 \nLabel=Strip\t808\tX=72775.96\ty=16873.45 \nLabel=Strip\t809\tX=72423.61\ty=16932.30 \nLabel=Strip\t810\tX=72770.14\ty=17030.50 \nLabel=Strip\t811\tX=72417.76\ty=17089.22 \nLabel=Strip\t812\tX=72764.26\ty=17187.54 \nLabel=Strip\t813\tX=72411.86\ty=17246.15 \nLabel=Strip\t814\tX=72758.32\ty=17344.59 \nLabel=Strip\t815\tX=72405.91\ty=17403.07 \nLabel=Strip\t816\tX=72752.33\ty=17501.63 \nLabel=Strip\t817\tX=72399.90\ty=17559.99 \nLabel=Strip\t818\tX=72746.29\ty=17658.67 \nLabel=Strip\t819\tX=72393.84\ty=17716.92 \nLabel=Strip\t820\tX=72740.19\ty=17815.71 \nLabel=Strip\t821\tX=72387.72\ty=17873.84 \nLabel=Strip\t822\tX=72734.04\ty=17972.75 \nLabel=Strip\t823\tX=72381.55\ty=18030.76 \nLabel=Strip\t824\tX=72727.84\ty=18129.79 \nLabel=Strip\t825\tX=72375.33\ty=18187.67 \nLabel=Strip\t826\tX=72721.58\ty=18286.83 \nLabel=Strip\t827\tX=72369.05\ty=18344.59 \nLabel=Strip\t828\tX=72715.27\ty=18443.87 \nLabel=Strip\t829\tX=72362.72\ty=18501.51 \nLabel=Strip\t830\tX=72708.90\ty=18600.90 \nLabel=Strip\t831\tX=72356.33\ty=18658.42 \nLabel=Strip\t832\tX=72702.48\ty=18757.93 \nLabel=Strip\t833\tX=72349.89\ty=18815.34 \nLabel=Strip\t834\tX=72696.01\ty=18914.97 \nLabel=Strip\t835\tX=72343.39\ty=18972.25 \nLabel=Strip\t836\tX=72689.48\ty=19072.00 \nLabel=Strip\t837\tX=72336.85\ty=19129.16 \nLabel=Strip\t838\tX=72682.90\ty=19229.03 \nLabel=Strip\t839\tX=72330.24\ty=19286.07 \nLabel=Strip\t840\tX=72676.26\ty=19386.06 \nLabel=Strip\t841\tX=72323.59\ty=19442.98 \nLabel=Strip\t842\tX=72669.57\ty=19543.09 \nLabel=Strip\t843\tX=72316.88\ty=19599.89 \nLabel=Strip\t844\tX=72662.82\ty=19700.12 \nLabel=Strip\t845\tX=72310.11\ty=19756.79 \nLabel=Strip\t846\tX=72656.03\ty=19857.14 \nLabel=Strip\t847\tX=72303.29\ty=19913.70 \nLabel=Strip\t848\tX=72649.17\ty=20014.17 \nLabel=Strip\t849\tX=72296.42\ty=20070.60 \nLabel=Strip\t850\tX=72642.27\ty=20171.19 \nLabel=Strip\t851\tX=72289.50\ty=20227.50 \nLabel=Strip\t852\tX=72635.30\ty=20328.21 \nLabel=Strip\t853\tX=72282.52\ty=20384.41 \nLabel=Strip\t854\tX=72628.29\ty=20485.23 \nLabel=Strip\t855\tX=72275.48\ty=20541.31 \nLabel=Strip\t856\tX=72621.22\ty=20642.25 \nLabel=Strip\t857\tX=72268.39\ty=20698.20 \nLabel=Strip\t858\tX=72614.10\ty=20799.27 \nLabel=Strip\t859\tX=72261.25\ty=20855.10 \nLabel=Strip\t860\tX=72606.92\ty=20956.28 \nLabel=Strip\t861\tX=72254.06\ty=21012.00 \nLabel=Strip\t862\tX=72599.69\ty=21113.30 \nLabel=Strip\t863\tX=72246.81\ty=21168.89 \nLabel=Strip\t864\tX=72592.41\ty=21270.31 \nLabel=Strip\t865\tX=72239.50\ty=21325.78 \nLabel=Strip\t866\tX=72585.07\ty=21427.32 \nLabel=Strip\t867\tX=72232.14\ty=21482.67 \nLabel=Strip\t868\tX=72577.67\ty=21584.33 \nLabel=Strip\t869\tX=72224.73\ty=21639.56 \nLabel=Strip\t870\tX=72570.23\ty=21741.34 \nLabel=Strip\t871\tX=72217.27\ty=21796.45 \nLabel=Strip\t872\tX=72562.73\ty=21898.35 \nLabel=Strip\t873\tX=72209.75\ty=21953.34 \nLabel=Strip\t874\tX=72555.17\ty=22055.35 \nLabel=Strip\t875\tX=72202.17\ty=22110.22 \nLabel=Strip\t876\tX=72547.56\ty=22212.36 \nLabel=Strip\t877\tX=72194.54\ty=22267.11 \nLabel=Strip\t878\tX=72539.90\ty=22369.36 \nLabel=Strip\t879\tX=72186.86\ty=22423.99 \nLabel=Strip\t880\tX=72532.18\ty=22526.36 \nLabel=Strip\t881\tX=72179.13\ty=22580.87 \nLabel=Strip\t882\tX=72524.41\ty=22683.36 \nLabel=Strip\t883\tX=72171.34\ty=22737.75 \nLabel=Strip\t884\tX=72516.58\ty=22840.36 \nLabel=Strip\t885\tX=72163.49\ty=22894.62 \nLabel=Strip\t886\tX=72508.70\ty=22997.35 \nLabel=Strip\t887\tX=72155.59\ty=23051.50 \nLabel=Strip\t888\tX=72500.77\ty=23154.35 \nLabel=Strip\t889\tX=72147.64\ty=23208.37 \nLabel=Strip\t890\tX=72492.78\ty=23311.34 \nLabel=Strip\t891\tX=72139.64\ty=23365.24 \nLabel=Strip\t892\tX=72484.74\ty=23468.33 \nLabel=Strip\t893\tX=72131.58\ty=23522.11 \nLabel=Strip\t894\tX=72476.65\ty=23625.32 \nLabel=Strip\t895\tX=72123.46\ty=23678.98 \nLabel=Strip\t896\tX=72468.50\ty=23782.31 \nLabel=Strip\t897\tX=72115.29\ty=23835.85 \nLabel=Strip\t898\tX=72460.30\ty=23939.29 \nLabel=Strip\t899\tX=72107.07\ty=23992.71 \nLabel=Strip\t900\tX=72452.04\ty=24096.28 \nLabel=Strip\t901\tX=72098.80\ty=24149.57 \nLabel=Strip\t902\tX=72443.73\ty=24253.26 \nLabel=Strip\t903\tX=72090.47\ty=24306.44 \nLabel=Strip\t904\tX=72435.36\ty=24410.24 \nLabel=Strip\t905\tX=72082.08\ty=24463.29 \nLabel=Strip\t906\tX=72426.94\ty=24567.22 \nLabel=Strip\t907\tX=72073.65\ty=24620.15 \nLabel=Strip\t908\tX=72418.47\ty=24724.19 \nLabel=Strip\t909\tX=72065.15\ty=24777.01 \nLabel=Strip\t910\tX=72409.94\ty=24881.17 \nLabel=Strip\t911\tX=72056.61\ty=24933.86 \nLabel=Strip\t912\tX=72401.36\ty=25038.14 \nLabel=Strip\t913\tX=72048.01\ty=25090.71 \nLabel=Strip\t914\tX=72392.72\ty=25195.11 \nLabel=Strip\t915\tX=72039.36\ty=25247.56 \nLabel=Strip\t916\tX=72384.03\ty=25352.08 \nLabel=Strip\t917\tX=72030.65\ty=25404.41 \nLabel=Strip\t918\tX=72375.29\ty=25509.04 \nLabel=Strip\t919\tX=72021.88\ty=25561.26 \nLabel=Strip\t920\tX=72366.49\ty=25666.01 \nLabel=Strip\t921\tX=72013.07\ty=25718.10 \nLabel=Strip\t922\tX=72357.64\ty=25822.97 \nLabel=Strip\t923\tX=72004.20\ty=25874.94 \nLabel=Strip\t924\tX=72348.74\ty=25979.93 \nLabel=Strip\t925\tX=71995.28\ty=26031.78 \nLabel=Strip\t926\tX=72339.77\ty=26136.89 \nLabel=Strip\t927\tX=71986.30\ty=26188.62 \nLabel=Strip\t928\tX=72330.76\ty=26293.85 \nLabel=Strip\t929\tX=71977.27\ty=26345.45 \nLabel=Strip\t930\tX=72321.69\ty=26450.80 \nLabel=Strip\t931\tX=71968.18\ty=26502.29 \nLabel=Strip\t932\tX=72312.57\ty=26607.75 \nLabel=Strip\t933\tX=71959.04\ty=26659.12 \nLabel=Strip\t934\tX=72303.40\ty=26764.70 \nLabel=Strip\t935\tX=71949.85\ty=26815.95 \nLabel=Strip\t936\tX=72294.17\ty=26921.65 \nLabel=Strip\t937\tX=71940.60\ty=26972.78 \nLabel=Strip\t938\tX=72284.88\ty=27078.60 \nLabel=Strip\t939\tX=71931.30\ty=27129.60 \nLabel=Strip\t940\tX=72275.54\ty=27235.54 \nLabel=Strip\t941\tX=71921.94\ty=27286.42 \nLabel=Strip\t942\tX=72266.15\ty=27392.48 \nLabel=Strip\t943\tX=71912.53\ty=27443.24 \nLabel=Strip\t944\tX=72256.71\ty=27549.42 \nLabel=Strip\t945\tX=71903.07\ty=27600.06 \nLabel=Strip\t946\tX=72247.21\ty=27706.36 \nLabel=Strip\t947\tX=71893.55\ty=27756.88 \nLabel=Strip\t948\tX=72237.65\ty=27863.29 \nLabel=Strip\t949\tX=71883.98\ty=27913.69 \nLabel=Strip\t950\tX=72228.04\ty=28020.23 \nLabel=Strip\t951\tX=71874.36\ty=28070.50 \nLabel=Strip\t952\tX=72218.38\ty=28177.16 \nLabel=Strip\t953\tX=71864.68\ty=28227.31 \nLabel=Strip\t954\tX=72208.67\ty=28334.09 \nLabel=Strip\t955\tX=71854.94\ty=28384.12 \nLabel=Strip\t956\tX=72198.90\ty=28491.01 \nLabel=Strip\t957\tX=71845.16\ty=28540.92 \nLabel=Strip\t958\tX=72189.07\ty=28647.93 \nLabel=Strip\t959\tX=71835.31\ty=28697.73 \nLabel=Strip\t960\tX=72179.19\ty=28804.85 \nLabel=Strip\t961\tX=71825.42\ty=28854.53 \nLabel=Strip\t962\tX=72169.26\ty=28961.77 \nLabel=Strip\t963\tX=71815.47\ty=29011.32 \nLabel=Strip\t964\tX=72159.27\ty=29118.69 \nLabel=Strip\t965\tX=71805.47\ty=29168.12 \nLabel=Strip\t966\tX=72149.23\ty=29275.60 \nLabel=Strip\t967\tX=71795.41\ty=29324.91 \nLabel=Strip\t968\tX=72139.14\ty=29432.51 \nLabel=Strip\t969\tX=71785.30\ty=29481.70 \nLabel=Strip\t970\tX=72128.99\ty=29589.42 \nLabel=Strip\t971\tX=71775.13\ty=29638.49 \nLabel=Strip\t972\tX=72118.79\ty=29746.33 \nLabel=Strip\t973\tX=71764.91\ty=29795.28 \nLabel=Strip\t974\tX=72108.53\ty=29903.23 \nLabel=Strip\t975\tX=71754.64\ty=29952.06 \nLabel=Strip\t976\tX=72098.22\ty=30060.14 \nLabel=Strip\t977\tX=71744.31\ty=30108.84 \nLabel=Strip\t978\tX=72087.86\ty=30217.03 \nLabel=Strip\t979\tX=71733.93\ty=30265.62 \nLabel=Strip\t980\tX=72077.44\ty=30373.93 \nLabel=Strip\t981\tX=71723.50\ty=30422.39 \nLabel=Strip\t982\tX=72066.97\ty=30530.82 \nLabel=Strip\t983\tX=71713.01\ty=30579.17 \nLabel=Strip\t984\tX=72056.44\ty=30687.72 \nLabel=Strip\t985\tX=71702.47\ty=30735.94 \nLabel=Strip\t986\tX=72045.86\ty=30844.60 \nLabel=Strip\t987\tX=71691.87\ty=30892.70 \nLabel=Strip\t988\tX=72035.23\ty=31001.49 \nLabel=Strip\t989\tX=71681.22\ty=31049.47 \nLabel=Strip\t990\tX=72024.54\ty=31158.37 \nLabel=Strip\t991\tX=71670.51\ty=31206.23 \nLabel=Strip\t992\tX=72013.80\ty=31315.25 \nLabel=Strip\t993\tX=71659.75\ty=31362.99 \nLabel=Strip\t994\tX=72003.00\ty=31472.13 \nLabel=Strip\t995\tX=71648.94\ty=31519.75 \nLabel=Strip\t996\tX=71992.15\ty=31629.01 \nLabel=Strip\t997\tX=71638.07\ty=31676.50 \nLabel=Strip\t998\tX=71981.24\ty=31785.88 \nLabel=Strip\t999\tX=71627.15\ty=31833.25 \nLabel=Strip\t1000\tX=71970.28\ty=31942.75 \nLabel=Strip\t1001\tX=71616.18\ty=31990.00 \nLabel=Strip\t1002\tX=71959.27\ty=32099.62 \nLabel=Strip\t1003\tX=71605.15\ty=32146.75 \nLabel=Strip\t1004\tX=71948.21\ty=32256.48 \nLabel=Strip\t1005\tX=71594.06\ty=32303.49 \nLabel=Strip\t1006\tX=71937.08\ty=32413.34 \nLabel=Strip\t1007\tX=71582.93\ty=32460.23 \nLabel=Strip\t1008\tX=71925.91\ty=32570.20 \nLabel=Strip\t1009\tX=71571.74\ty=32616.97 \nLabel=Strip\t1010\tX=71914.68\ty=32727.06 \nLabel=Strip\t1011\tX=71560.49\ty=32773.71 \nLabel=Strip\t1012\tX=71903.40\ty=32883.91 \nLabel=Strip\t1013\tX=71549.19\ty=32930.44 \nLabel=Strip\t1014\tX=71892.06\ty=33040.76 \nLabel=Strip\t1015\tX=71537.84\ty=33087.17 \nLabel=Strip\t1016\tX=71880.67\ty=33197.61 \nLabel=Strip\t1017\tX=71526.43\ty=33243.89 \nLabel=Strip\t1018\tX=71869.23\ty=33354.45 \nLabel=Strip\t1019\tX=71514.97\ty=33400.62 \nLabel=Strip\t1020\tX=71857.73\ty=33511.30 \nLabel=Strip\t1021\tX=71503.46\ty=33557.34 \nLabel=Strip\t1022\tX=71846.17\ty=33668.13 \nLabel=Strip\t1023\tX=71491.89\ty=33714.05 \nLabel=Strip\t1024\tX=71834.57\ty=33824.97 \nLabel=Strip\t1025\tX=71480.27\t
